vi "Read Voltage From Channel.vi"(8 "error in (no error)":errorcluster, 10 "Channel":u8, 11 "IRead Voltage Multichannel in":refnum<class "IRead Voltage from Channel.lvclass">) -> (0 "error out":errorcluster, 2 "Voltage":dbl format="%#_g V", 3 "IRead Voltage Multichannel out":refnum<class "IRead Voltage from Channel.lvclass">)   [LabVIEW 2023, in "HAL Interfaces.lvlib" / "IRead Voltage from Channel.lvclass"]
uses:
  IRead Voltage from Channel.lvclass
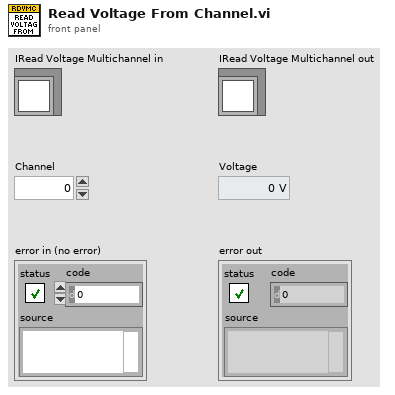
[diagram p1: front panel]
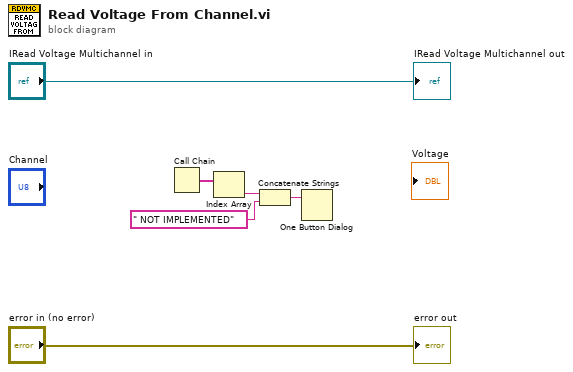
[diagram p0: block diagram]
diagram:
  n1 = Call Chain() -> (call chain=w4:string[])
  n2 = Index Array(array=w4) -> (element=w2:string)  [unwired: 1 in]
  n3 = Concatenate Strings(w2, " NOT IMPLEMENTED" ("string")) -> (w3:string)
  n4 = One Button Dialog(message=w3) -> ()  [unwired: 1 in, 1 out]
  "error out" <- "error in (no error)"
  "IRead Voltage Multichannel out" <- "IRead Voltage Multichannel in"
